vi "ATM_FP.Consolidate_Response_msg.vi"(0 "ResponseMessage":string) -> (14 "ResponseMessage (duplicate)":string, 15 "returnParameter":string, 16 "confirmationMsg":string, 17 "confirmationCode":string, 18 "responseOK?":bool, 19 "Match":bool)   [LabVIEW 2020]
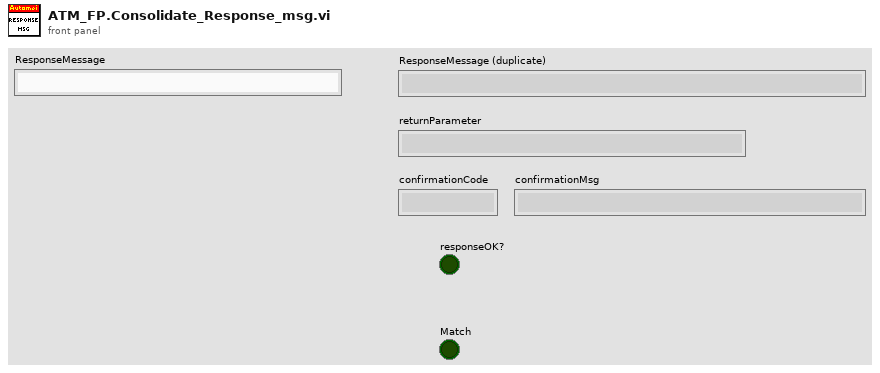
[diagram p1: front panel]
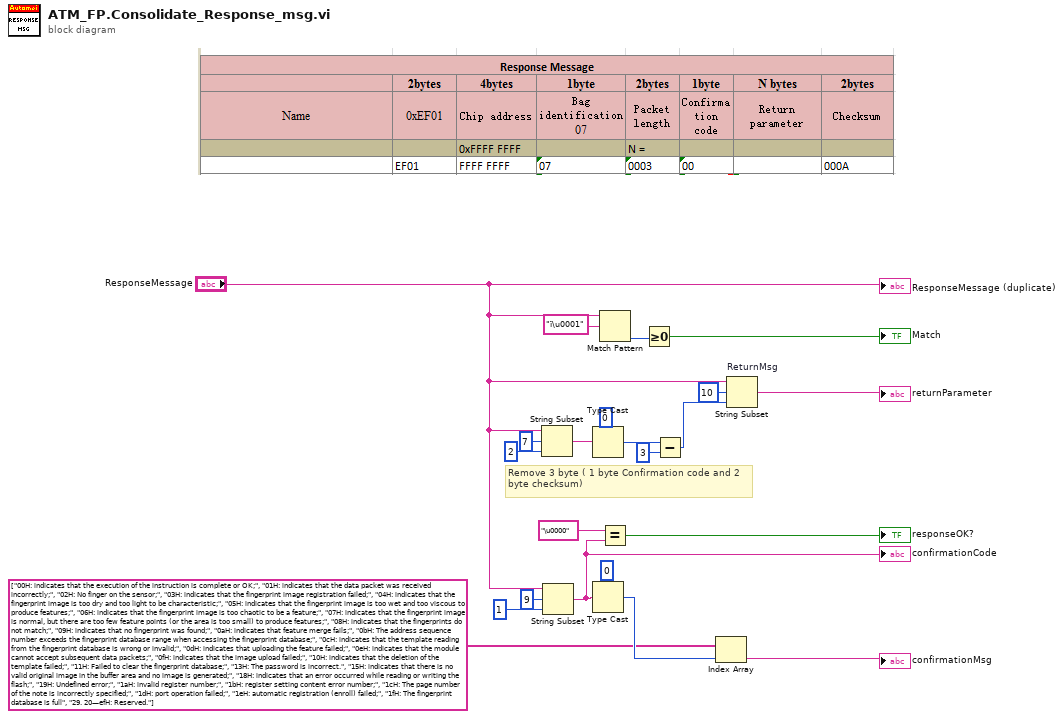
[diagram p0: block diagram]
diagram:
  # "Remove 3 byte ( 1 byte Confirmation code and 2 byte checksum)"
  n1 = String Subset(string="ResponseMessage", offset (0)=7, length (rest)=2 ("length (rest)")) -> (substring=w6:string)
  n2 = String Subset(string="ResponseMessage", offset (0)=9, length (rest)=1 ("length (rest)")) -> (substring=w16:string)
  "confirmationCode" <- w16
  n3 = Type Cast(type=u16 0, x=w6) -> (*(type *) &x=w8:u16)
  n4 = Type Cast(type=u8 0, x=w16) -> (*(type *) &x=w17:u8)
  n5 = Match Pattern(string="ResponseMessage", regular expression="ï\u0001") -> (offset past match=w21:i32)  [unwired: 1 in, 3 out]
  n6 = Equal?(x="\u0000", y=w16) -> (x = y?=→"responseOK?":bool)
  n7 = Greater Or Equal To 0?(x=w21) -> (x >= 0?=→"Match":bool)
  n8 = Subtract(x=w8, y=u16 3) -> (x-y=w4:u16)
  n9 = Index Array(array=string[] ["00H: indicates that the execution of the instruction is complete or OK;", "01H: indicates that the data packet was received incorrectly;", "02H: No finger on the sensor;", "03H: indicates that the fingerprint image registration failed;", "04H: indicates that the fingerprint image is too dry and too light to be characteristic;", "05H: indicates that the fingerprint image is too wet and too viscous to produce features;", "06H: indicates that the fingerprint image is too chaotic to be a feature;", "07H: indicates that the fingerprint image is normal, but there are too few feature points (or the area is too small) to produce features;", "08H: indicates that the fingerprints do not match;", "09H: indicates that no fingerprint was found;", "0aH: indicates that feature merge fails;", "0bH: The address sequence number exceeds the fingerprint database range when accessing the fingerprint database;", "0cH: indicates that the template reading from the fingerprint database is wrong or invalid;", "0dH: indicates that uploading the feature failed;", "0eH: indicates that the module cannot accept subsequent data packets;", "0fH: indicates that the image upload failed;", "10H: indicates that the deletion of the template failed;", "11H: Failed to clear the fingerprint database;", "13H: The password is incorrect.", "15H: indicates that there is no valid original image in the buffer area and no image is generated;", "18H: indicates that an error occurred while reading or writing the flash;", "19H: Undefined error;", "1aH: invalid register number;", "1bH: register setting content error number;", "1cH: The page number of the note is incorrectly specified;", "1dH: port operation failed;", "1eH: automatic registration (enroll) failed;", "1fH: The fingerprint database is full", "29. 20—efH: Reserved."], index=w17) -> (element=→"confirmationMsg":string)
  n10 = String Subset "ReturnMsg"(string="ResponseMessage", offset (0)=10, length (rest)=w4) -> (substring=→"returnParameter":string)
  "ResponseMessage (duplicate)" <- "ResponseMessage"
